vi "PXIe-433x Inline RT Driver VI.vi"(7 "Operation":T1, 11 "Device Reference in":T2 format="%.0x") -> (0 "Error Code":i32)   [LabVIEW 2011, in "PXIe-433x Custom Device.lvlib"]
uses:
  PXIe-433x Custom Device.lvlib
  <vilib>/NI Veristand/Custom Device API/Custom Device Item Ref.ctl
  <vilib>/NI Veristand/Custom Device API/Hardware Interface Driver VI Operation.ctl
  Inline RT Data.ctl
  <vilib>/NI Veristand/Custom Device API/Block Data Reference.ctl
  <vilib>/NI Veristand/Custom Device API/Data Reference.ctl
  <vilib>/NI Veristand/Custom Device API/Data Access Type.ctl
  Global.vi
  <vilib>/NI Veristand/Custom Device Tools/Custom Device Utility Library/NI VeriStand - Search for All Items by GUID.vi
  <vilib>/NI Veristand/Custom Device API/Get Item Property (Boolean).vi
  <vilib>/DAQmx/configure/timing.llb/DAQmx Timing (Sample Clock).vi
  <vilib>/DAQmx/miscellaneous.llb/DAQmx Fill In Error Info.vi
  <vilib>/NI Veristand/Custom Device API/Global Data Refs.vi
  <vilib>/NI Veristand/Custom Device API/Custom Device API.lvlib
  <vilib>/NI Veristand/Custom Device Tools/Custom Device Utility Library/Custom Device Utility Library.lvlib
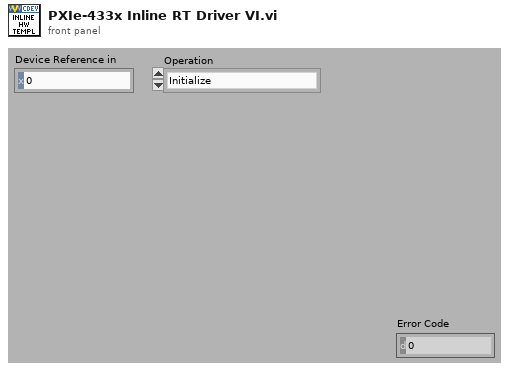
[diagram p1: front panel]
types:
  T1 = typedef "Custom Device API.lvlib/Hardware Interface Driver VI Operation.ctl" = enum16{"Initialize", "Start", "Read Data from HW", "Write Data to HW", "Close"}
  T2 = typedef "Custom Device API.lvlib/Custom Device Item Ref.ctl" = u64
  T3 = typedef "PXIe-433x Custom Device.lvlib/Inline RT Data.ctl" = cluster{"task":refnum<k21>, "BD Refs":T4[], "Vals":dbl[], "Run?":bool}
  T4 = typedef "Custom Device API.lvlib/Block Data Reference.ctl" = cluster{"Data Reference":T5, "Offset":i32, "Length":i32}
  T5 = typedef "Custom Device API.lvlib/Data Reference.ctl" = i32
  T6 = typedef "Custom Device API.lvlib/Data Access Type.ctl" = enum16{"Read", "Write"}
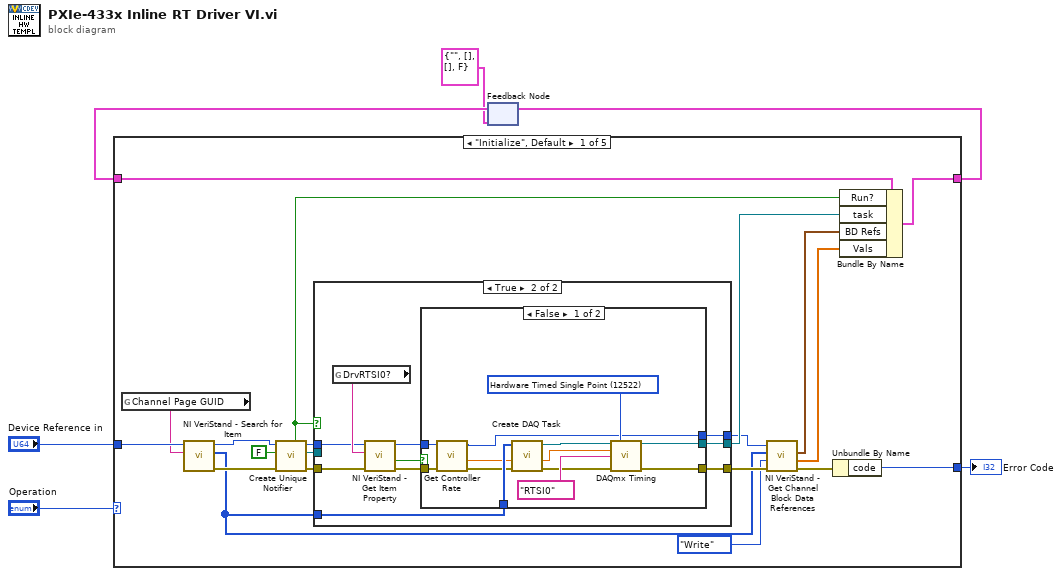
[diagram p0: block diagram]
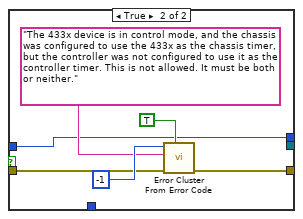
[diagram p3: hidden frame]
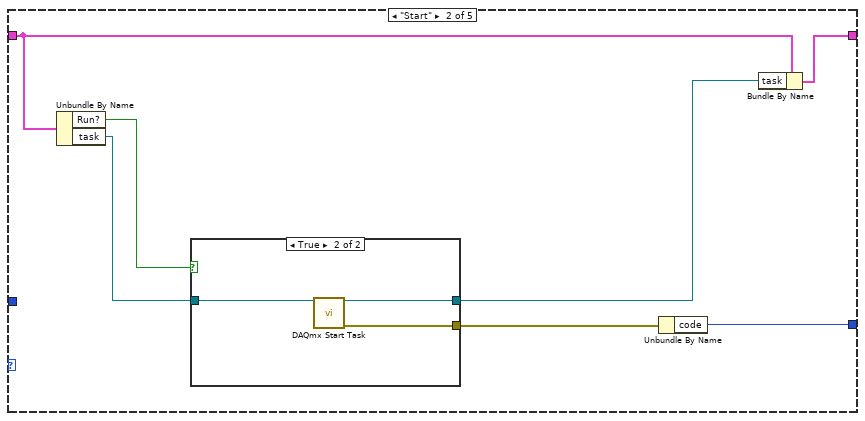
[diagram p4: hidden frame]
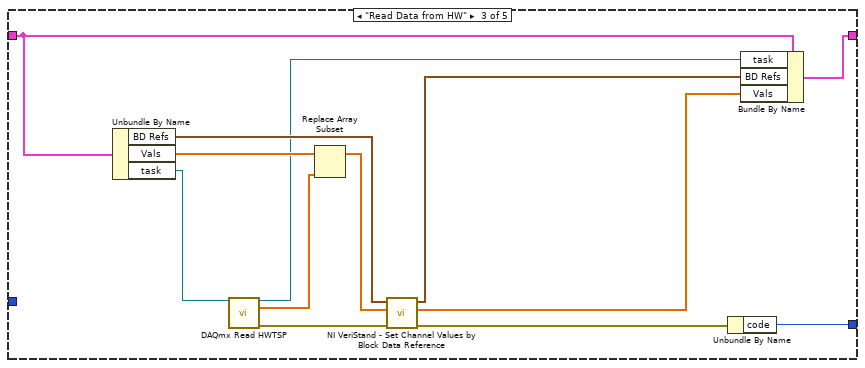
[diagram p6: hidden frame]
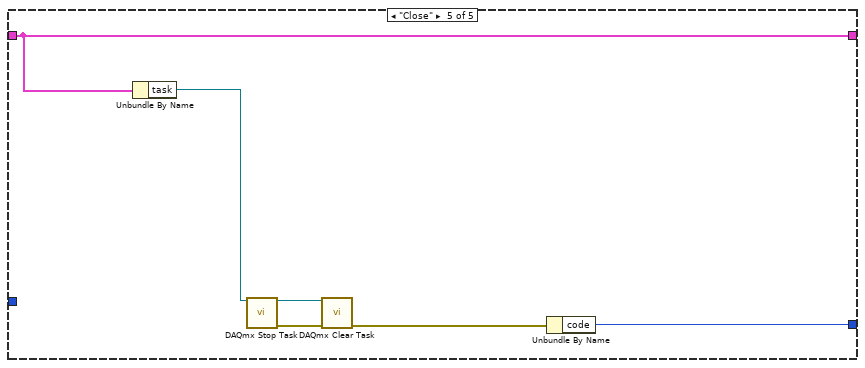
[diagram p8: hidden frame]
diagram:
  n1 = feedback #1(T3 {"task"="", "BD Refs"=[], "Vals"=[], "Run?"=FALSE} ("RT Data")) -> (w4:T3)
  n2 = case shown="\"Initialize\", Default" "Operation" {
    tunnel: [w9 w63 w80 w83 w84] -> w5
    tunnel: w4 -> [w21 w64 w81 w83 w84]
    tunnel: "Device Reference in" -> [w18 _ _ _ _]
    tunnel: [w22 w65 w82 _ w86] -> w2
    frame "Initialize", Default {
      n3 = global read "Global.vi" "Channel Page GUID"() -> (w17:string)
      n4 = call-poly <vilib>:"NI VeriStand - Search for Item.vi"("Item GUID"=w17, "Section Ref in"=w18) -> ("error out"=w19:errorcluster, "Item Refs"=w8:T2[], "Section Ref out"=w16:T2)  [unwired: 6 in, 1 out]
      n5 = call "Create Unique Notifier.vi"("error in"=w19, "Send? (T)"=FALSE, "Device Ref"=w16) -> ("error out"=w25:errorcluster, "DAQ task received"=w24:refnum<k21>, "Device Ref dup"=w23:T2, "created new?"=w7:bool)  [unwired: 5 in]
      n6 = case shown="True" w7 {
        tunnel: w25 -> [w28 w32]
        tunnel: w24 -> [w29 _]
        tunnel: w23 -> [w27 w38]
        tunnel: [w28 w31] -> w15
        tunnel: [w29 w30] -> w20
        tunnel: w8 -> [_ w34]
        tunnel: [w27 w33] -> w13
        frame False {
        }
        frame True {
          n7 = global read "Global.vi" "DrvRTSI0?"() -> (w39:string)
          n8 = call-poly <vilib>:"NI VeriStand - Get Item Property.vi"("error in (no error)"=w32, "Property Name"=w39, "Item Ref in"=w38) -> ("error out"=w37:errorcluster, "Value"=w36:bool, "Item Ref out"=w35:T2)  [unwired: 5 in, 1 out]
          n9 = case shown="False" w36 {
            tunnel: w37 -> [w44 w56]
            tunnel: [w47 w54] -> w31
            tunnel: [w46 _] -> w30
            tunnel: w35 -> [w43 w53]
            tunnel: w34 -> [w45 _]
            tunnel: [w40 w53] -> w33
            frame False {
              w50 = 12522 items=["Finite Samples"=10178, "Continuous Samples"=10123, "Hardware Timed Single Point"=12522] ("sample mode")
              n10 = call "Get Controller Rate.vi"("error in (no error)"=w44, "Device Reference In"=w43) -> ("error out"=w42:errorcluster, "Rate in Hz"=w41:dbl, "Device Reference dup"=w40:T2)  [unwired: 6 in, 1 out]
              n11 = call "Create DAQ Task.vi"("error in"=w42, "User provided rate"=w41, "Channels"=w45) -> ("error out"=w49:errorcluster, "Actual rate"=w48:dbl, "task out"=w51:refnum<k21>)  [unwired: 6 in]
              n12 = call-poly <vilib>:"DAQmx Timing.vi"("task/channels in"=w51, "sample mode"=w50, "rate"=w48, "source"=tag "RTSI0" ("output terminal"), "error in"=w49) -> ("task out"=w46:refnum<k21>, "error out"=w47:errorcluster)  [unwired: 9 in]
            }
            frame True {
              n13 = call <vilib>:"Error Cluster From Error Code.vi"("show call chain? (False)"=TRUE, "error in (no error)"=w56, "error message (\"\")"="The 433x device is in control mode, and the chassis was configured to use the 433x as the chassis timer, but the controller was not configured to use it as the controller timer. This is not allowed. It must be both or neither." ("error message (\"\")"), "error code (0)"=-1) -> ("error out"=w54:errorcluster)  [unwired: 5 in]
            }
          }
        }
      }
      n14 = call <vilib>:"NI VeriStand - Get Channel Block Data References.vi"("error in (no error)"=w15, "Access"=Data_Access_Type."Write", "Channel Refs"=w8, "Device Ref in"=w13) -> ("error out"=w10:errorcluster, "Values Array"=w11:dbl[], "Block Data Refs"=w12:T4[])  [unwired: 4 in, 1 out]
      n15 = Unbundle By Name(w10) -> ("code"=w22:i32)
      n16 = Bundle By Name(cluster=w21, "Run?"=w7, "task"=w20, "BD Refs"=w12, "Vals"=w11) -> (w9:T3)
    }
    frame "Start" {
      n17 = Unbundle By Name(w64) -> ("Run?"=w62:bool, "task"=w61:refnum<k21>)
      n18 = case shown="True" w62 {
        tunnel: w61 -> [w66 w69]
        tunnel: [_ w68] -> w60
        tunnel: [w66 w67] -> w59
        frame False {
        }
        frame True {
          n19 = call <vilib>:"DAQmx Start Task.vi"("task/channels in"=w69) -> ("task out"=w67:refnum<k21>, "error out"=w68:errorcluster)  [unwired: 13 in]
        }
      }
      n20 = Unbundle By Name(w60) -> ("code"=w65:i32)
      n21 = Bundle By Name(cluster=w64, "task"=w59) -> (w63:T3)
    }
    frame "Read Data from HW" {
      n22 = Unbundle By Name(w81) -> ("BD Refs"=w79:T4[], "Vals"=w74:dbl[], "task"=w78:refnum<k21>)
      n23 = call "DAQmx Read HWTSP.vi"("task/channels in"=w78) -> ("task out"=w71:refnum<k21>, "data"=w72:dbl[], "error out"=w77:errorcluster)  [unwired: 12 in]
      n24 = Replace Array Subset(array=w74, new element=w72) -> (w73:dbl[])  [unwired: 1 in]
      n25 = call <vilib>:"NI VeriStand - Set Channel Values by Block Data Reference.vi"("error in (no error)"=w77, "Values Array in"=w73, "Block Data Ref"=w79) -> ("error out"=w76:errorcluster, "Values Array out"=w70:dbl[], "Block Data Ref dup"=w75:T4[])  [unwired: 6 in]
      n26 = Unbundle By Name(w76) -> ("code"=w82:i32)
      n27 = Bundle By Name(cluster=w81, "task"=w71, "BD Refs"=w75, "Vals"=w70) -> (w80:T3)
    }
    frame "Write Data to HW" {
    }
    frame "Close" {
      n28 = Unbundle By Name(w84) -> ("task"=w89:refnum<k21>)
      n29 = call <vilib>:"DAQmx Stop Task.vi"("task/channels in"=w89) -> ("task out"=w87:refnum<k21>, "error out"=w88:errorcluster)  [unwired: 13 in]
      n30 = call <vilib>:"DAQmx Clear Task.vi"("task in"=w87, "error in"=w88) -> ("error out"=w85:errorcluster)  [unwired: 13 in]
      n31 = Unbundle By Name(w85) -> ("code"=w86:i32)
    }
  }
  "Error Code" <- w2
  n32 = feedback-in #1(w5) -> ()
